vi "Initialize.vi"(2 "XRef":refnum<vi>) -> (1 "State Out":T1={"Input Type"=variant(dbl 0.0), "Width"=0, "Typedef Name"="", "Value Type"=variant, "Selection"=0, "Options"=[], "Selections"=[], "Display Selections"=[], "Element Names"=[], "Typedef Name Width"=0, "Display Selection Width"=[], "Code Generated"=FALSE})   [LabVIEW 2015, in "Read-Write-Signals.xnode"]
doc: "This ability VI is called when your XNode is first dropped. It is used to specify your initial state.\n\nDefault behavior: Intialize state to default defaults (usually zero-initialized).\n\nThis ability does not provide UI and OS messages are not handled.\n\nSee also: Copy"
uses:
  Read-Write-Signals.xnode
  State.ctl
  Read-Write-Signals Item.ctl
  Read-Write-Signals Sub Item.ctl
  Read-Write-Signals Sub Item Type.ctl
  Read-Write-Signals Selection.ctl
  Read-Write-Signals Display Selection.ctl
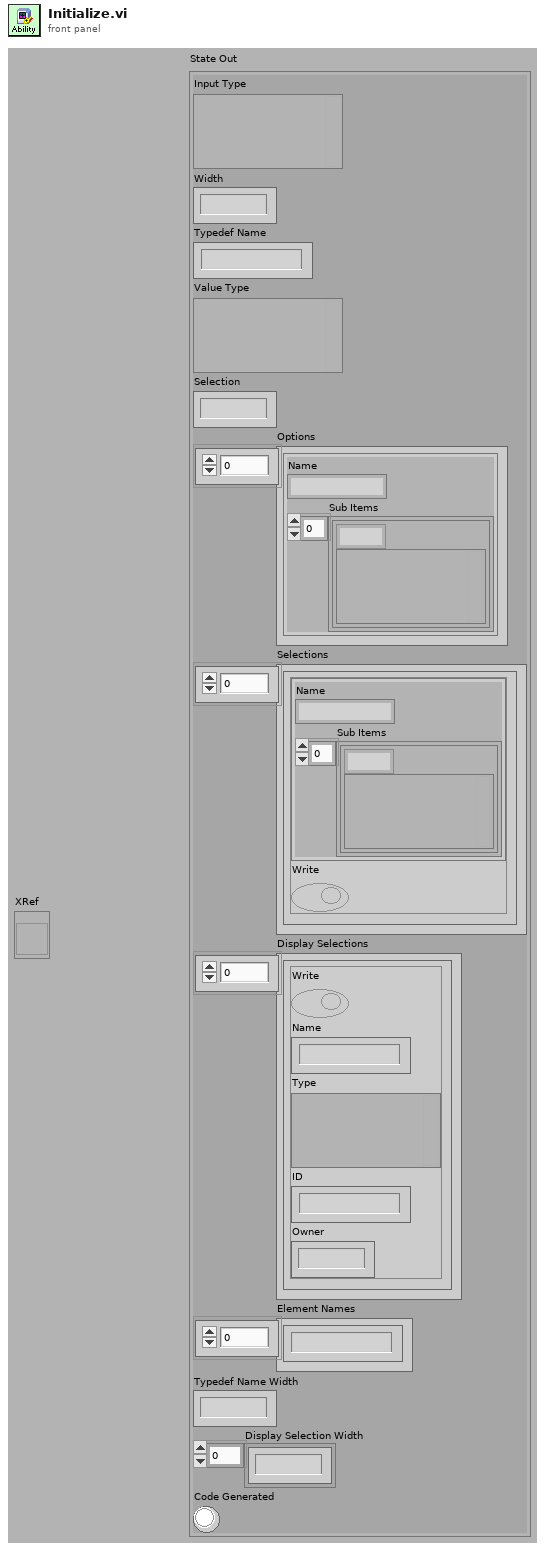
[diagram p1: front panel]
types:
  T1 = typedef "Read-Write-Signals.xnode/State.ctl" = cluster{"Input Type":variant, "Width":i32, "Typedef Name":string, "Value Type":variant, "Selection":i32, "Options":T2[], "Selections":T5[], "Display Selections":T6[], "Element Names":string[], "Typedef Name Width":i32, "Display Selection Width":i32[], "Code Generated":bool}
  T2 = typedef "Read-Write-Signals Item.ctl" = cluster{"Name":string, "Sub Items":T3[]}
  T3 = typedef "Read-Write-Signals Sub Item.ctl" = cluster{"Type":T4, "Value":variant}
  T4 = typedef "Read-Write-Signals Sub Item Type.ctl" = enum8{"Cluster Element", "Array Element", "Subarray"}
  T5 = typedef "Read-Write-Signals Selection.ctl" = cluster{"Item":T2, "Write":bool}
  T6 = typedef "Read-Write-Signals Display Selection.ctl" = cluster{"Write":bool, "Name":string, "Type":variant, "ID":string, "Owner":i32}
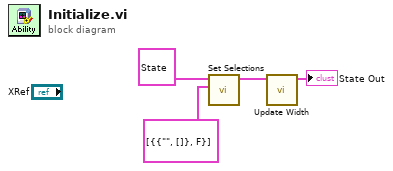
[diagram p0: block diagram]
diagram:
  n1 = call "Set Selections.vi"("Selections"=T5[] [{"Item"={"Name"="", "Sub Items"=[]}, "Write"=FALSE}], "State in"=T1 {"Input Type"=variant, "Width"=0, "Typedef Name"="", "Value Type"=variant, "Selection"=0, "Options"=[], "Selections"=[], "Display Selections"=[], "Element Names"=[], "Typedef Name Width"=0, "Display Selection Width"=[], "Code Generated"=FALSE} ("State")) -> ("State out"=w2:T1)  [unwired: 8 in, 1 out]
  n2 = call "Update Width.vi"("State in in"=w2) -> ("State out"=→"State Out":T1)  [unwired: 10 in]
